vi "脉冲生成_基于时钟滴答_单脉冲.vi"() -> ()   [LabVIEW 2013]
uses:
  <userlib>/ArtDAQ/_SubVI/ArtDAQ_CreateCOPulseChanTicks.vi
  <userlib>/ArtDAQ/_SubVI/ArtDAQ_CfgDigEdgeStartTrig.vi
panel:
  in  "时钟滴答源":string="/Dev1/PFI1"
  in  "TriggerMode":enum32{"No Trigger", "DigStartTrig"}(tab)
  in  "触发边沿":i32(ring)=10280 items=["上升"=10280, "下降"=10171]
  in  "触发源":string(combo)="/Dev1/PFI2"
  in  "Stop":bool
  in  "计数器":string="Dev1/ctr0"
  in  "高滴答数":i32=100
  in  "低滴答数":i32=100
  out "错误输出":errorcluster
  # "通道属性"
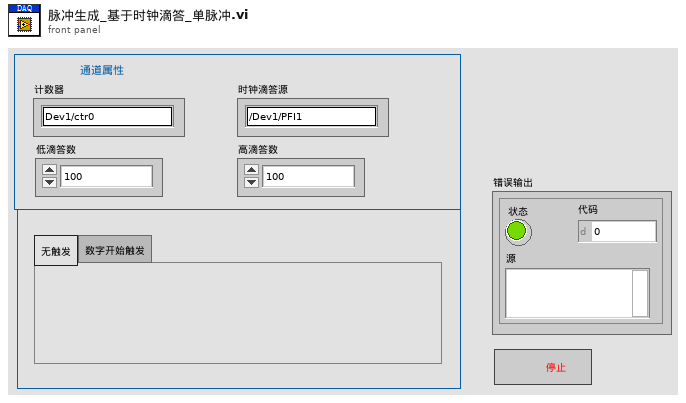
[diagram p1: front panel]
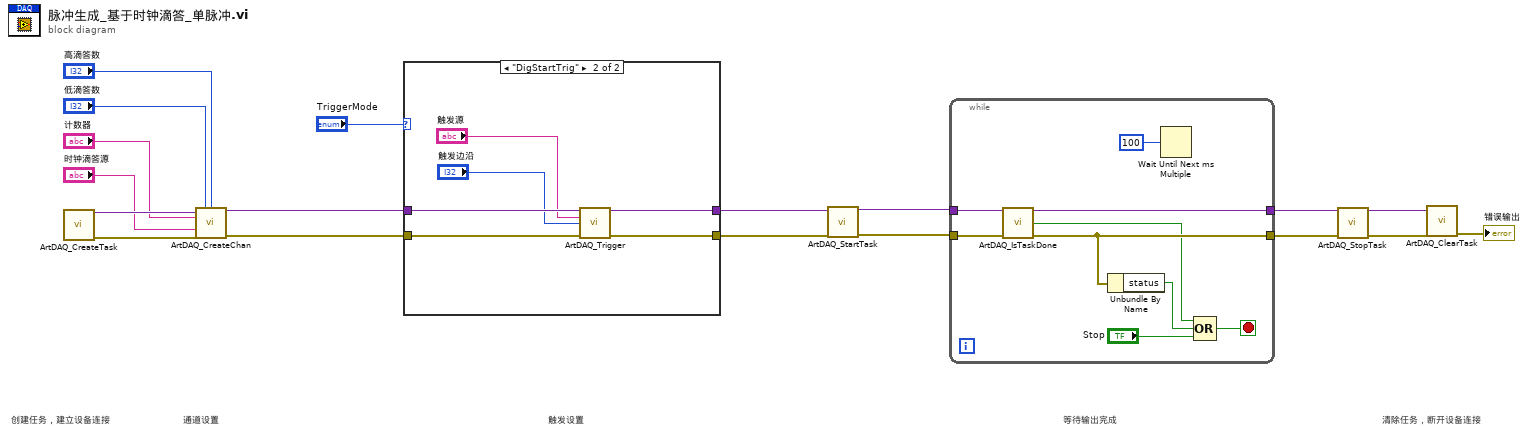
[diagram p0: block diagram]
diagram:
  # "创建任务，建立设备连接"
  # "通道设置"
  # "触发设置"
  # "等待输出完成"
  # "清除任务，断开设备连接"
  n1 = call <userlib>:"ArtDAQ_CreateTask.vi"() -> ("任务句柄"=w18:variant, "错误输出"=w17:errorcluster)  [unwired: 14 in]
  n2 = call-poly <userlib>:"ArtDAQ_CreateChan.vi"("任务句柄"=w18, "低时钟嘀嗒"="低滴答数", "高时钟嘀嗒"="高滴答数", "计数器"="计数器", "时钟嘀嗒源"="时钟滴答源", "错误输入"=w17) -> ("任务句柄"=w2:variant, "错误输出"=w1:errorcluster)  [unwired: 8 in]
  n3 = case shown="\"DigStartTrig\"" "TriggerMode" {
    tunnel: w2 -> [w20 w26]
    tunnel: [w20 w25] -> w8
    tunnel: [w19 w24] -> w6
    tunnel: w1 -> [w19 w23]
    frame "No Trigger", Default {
    }
    frame "DigStartTrig" {
      n4 = call-poly <userlib>:"ArtDAQ_Trigger.vi"("任务句柄"=w26, "触发源"="触发源", "边沿"="触发边沿", "错误输入"=w23) -> ("任务句柄"=w25:variant, "错误输出"=w24:errorcluster)  [unwired: 10 in]
    }
  }
  n5 = call <userlib>:"ArtDAQ_StartTask.vi"("任务句柄"=w8, "错误输入"=w6) -> ("任务句柄"=w7:variant, "错误输出"=w5:errorcluster)  [unwired: 12 in]
  n6 = while {
    tunnel: [w35] -> w16
    tunnel: [w34] -> w14
    tunnel: w7 -> [w31]
    tunnel: w5 -> [w30]
    stop <- w29 stop-if-true
    n7 = call <userlib>:"ArtDAQ_IsTaskDone.vi"("任务句柄"=w31, "错误输入"=w30) -> ("任务句柄"=w35:variant, "完成任务？"=w27:bool, "错误输出"=w34:errorcluster)  [unwired: 11 in]
    n8 = Unbundle By Name(w34) -> ("status"=w33:bool)
    n9 = Wait Until Next ms Multiple(millisecond multiple=u32 100 ("毫秒倍数")) -> ()  [unwired: 1 out]
    n10 = Compound Arithmetic op=OR(w27, w33, "Stop") -> (w29:bool)
  }
  n11 = call <userlib>:"ArtDAQ_StopTask.vi"("任务句柄"=w16, "错误输入"=w14) -> ("任务句柄"=w15:variant, "错误输出"=w13:errorcluster)  [unwired: 12 in]
  n12 = call <userlib>:"ArtDAQ_ClearTask.vi"("任务句柄"=w15, "错误输入"=w13) -> ("错误输出"=→"错误输出":errorcluster)  [unwired: 13 in]
